vi "Generate Bitfile Path.vi"() -> (0 "System Definition path":path)   [LabVIEW 2019, in "Max Nr of Scalar Channels.lvclass"]
uses:
  Max Nr of Scalar Channels.lvclass
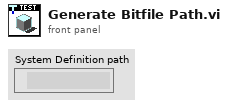
[diagram p1: front panel]
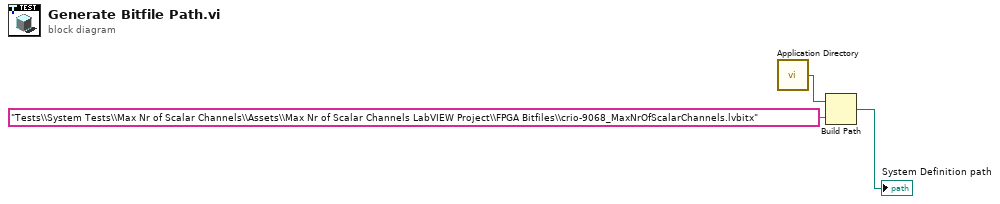
[diagram p0: block diagram]
diagram:
  n1 = call <vilib>:"Application Directory.vi"() -> ("Application Directory"=w1:path)
  n2 = Build Path(base path=w1, name or relative path="Tests\\System Tests\\Max Nr of Scalar Channels\\Assets\\Max Nr of Scalar Channels LabVIEW Project\\FPGA Bitfiles\\crio-9068_MaxNrOfScalarChannels.lvbitx") -> (appended path=→"System Definition path":path)
